vi "Conditionally Obtain Buffer.vi"(8 "error in (no error)":errorcluster, 11 "buffer":refnum<data-value>) -> (0 "error out":errorcluster, 3 "buffer":refnum<data-value>)   [LabVIEW 2017, in "Waveforms (N Ch).lvclass"]
doc: "Use this VI to conditionally create a DVR to a new buffer. This VI performs implicit buffer creation such that simple single writer, single reader operations can be performed without requiring Obtain Buffer.vi"
uses:
  <vilib>/addons/_NISVFA/_Shared subVIs/Data Objects/Waveforms (DBL)/Waveforms (N Ch).lvclass
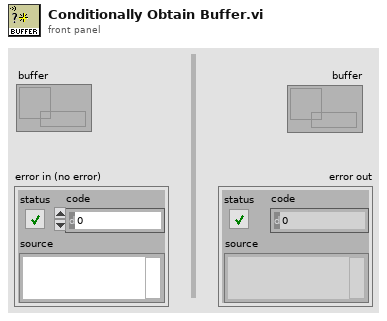
[diagram p1: front panel]
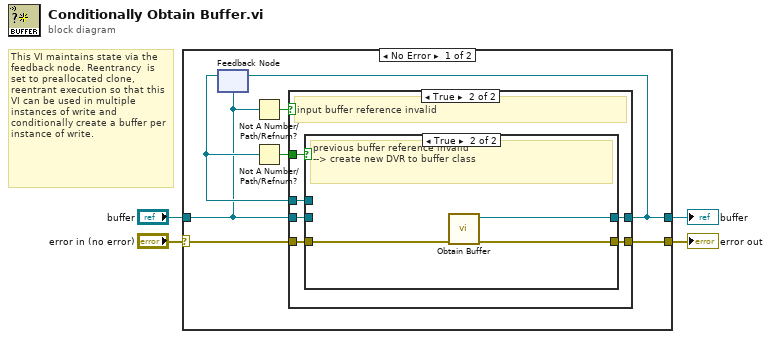
[diagram p0: block diagram]
diagram:
  # "This VI maintains state via the feedback node. Reentrancy  is set to preallocated clone, reentrant execution so that this VI can be used in multiple instances of write and conditionally create a buffer per instance of write."
  n1 = case shown="No Error" "error in (no error)" {
    selector: "error in (no error)" -> [w5 w26]
    tunnel: "buffer" -> [w7 w25]
    tunnel: [w11 w26] -> w2
    tunnel: [w6 w25] -> w1
    frame No Error {
      n2 = feedback #1(w7) -> (w8:refnum<data-value>)
      n3 = Not A Number/Path/Refnum?(number/path/refnum=w7) -> (NaN/Path/Refnum?=w9:bool)
      n4 = Not A Number/Path/Refnum?(number/path/refnum=w8) -> (NaN/Path/Refnum?=w10:bool)
      n5 = case shown="True" w9 {
        tunnel: [w13 w19] -> w11
        tunnel: [w12 w15] -> w6
        tunnel: w5 -> [w13 w18]
        tunnel: w10 -> [_ w17]
        tunnel: w8 -> [_ w16]
        tunnel: w7 -> [w12 w14]
        frame False {
          # "input buffer (DVR) is valid reference"
        }
        frame True {
          # "input buffer reference invalid"
          n6 = case shown="True" w17 {
            tunnel: w18 -> [w21 w24]
            tunnel: [w21 w23] -> w19
            tunnel: w16 -> [w20 _]
            tunnel: [w20 w22] -> w15
            tunnel: w14 -> [_ _]
            frame False {
              # "previous buffer reference valid, use it"
            }
            frame True {
              # "previous buffer reference invalid\n--> create new DVR to buffer class"
              n7 = call <vilib>:"Obtain Buffer.vi"("error in (no error)"=w24) -> ("error out"=w23:errorcluster, "buffer out"=w22:refnum<data-value>)  [unwired: 9 in]
            }
          }
        }
      }
      n8 = feedback-in #1(w6) -> ()
    }
    frame Error {
    }
  }
  "buffer" <- w1
  "error out" <- w2
